vi "Get Actual Voltage.vi"(8 "error in":errorcluster, 11 "TEC 1090 in":refnum<class "Meerstetter TEC.lvclass">) -> (0 "error out":errorcluster, 2 "Number":sgl=92.92 format="%.10f", 3 "TEC 1090 out":refnum<class "Meerstetter TEC.lvclass">)   [LabVIEW 2014, in "Meerstetter Lib.lvlib" / "Meerstetter TEC.lvclass"]
uses:
  Meerstetter TEC.lvclass
  Controls/Read Parameters.ctl
  reusable/Session APIs/Serial/Serial Session.lvclass
  Meerstetter TEC.lvclass/Meerstetter TEC.ctl
  reusable/Session APIs/Serial/Public/Asynchronous Write.vi
  reusable/Session APIs/Serial/Public/Asynchronous Read.vi
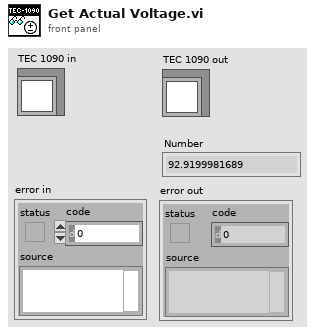
[diagram p1: front panel]
types:
  T1 = typedef "Read Parameters.ctl" = u16
  T2 = typedef "Session - Root.lvclass/Session Handle.ctl" = refnum<data-value>
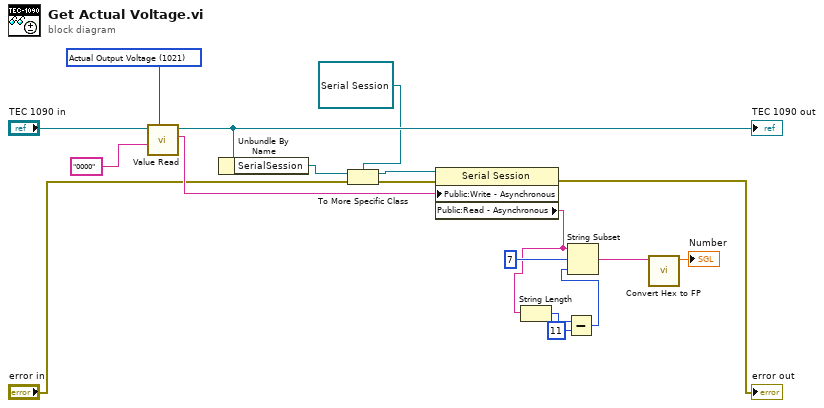
[diagram p0: block diagram]
diagram:
  w17 = T1 1021 items=["Device Type"=100, "Hardware Version"=101, "Serial Number"=102, "Firmware Version"=103, "Device Status"=104, "Error Number"=105, "Error Instance"=106, "Error Parameter"=107, "Save Data to Flash"=108, "Flash Status"=109, "Object Temperature"=1000, "Sink Temperature"=1001, "Target Obj Temperature"=1010, "Nominal Obj Temperature"=1011, "Thermal Power Mod Current"=1012, "Actual Output Current"=1020, "Actual Output Voltage"=1021, "Relative Cooling Power"=1100, "Nominal Fan Speed"=1101, "Actual Fan Speed"=1102, "Fan PWM Level"=1103, "PID Lower Limitation"=1030, "PID Upper Limitation"=1031, "PID Control Variable"=1032, "Obj Sensor Raw ADC Val"=1040, "Sink Sensor Raw ADC Val"=1041, "Object Sensor Resistance"=1042, "Sink Sensor Resistance"=1043, "Driver Input Voltage"=1060, "10V Internal Supply"=1061, "3.3V Internal Supply"=1062, "Base Plate Temperature"=1063, "Error Number"=1070, "Error Instance"=1071, "Error Parameter"=1072, "Temperature is Stable"=1200] ("Read Values")
  n1 = call "Value Read.vi"("Read Values"=w17, "Sequence"="0000", "TEC 1090"="TEC 1090 in") -> ("hex integer string"=w4:string, "TEC 1091"=w9:refnum<class "Meerstetter TEC.lvclass">)  [unwired: 7 in]
  "TEC 1090 out" <- w9
  n2 = Unbundle By Name(w9) -> ("SerialSession"=w8:T2)
  n3 = To More Specific Class(target class=refnum<data-value> refnum, reference=w8, error in="error in") -> (specific class reference=w6:refnum<data-value>, error out=w2:errorcluster)
  n4 = property class="Serial Session"(reference=w6, error in=w2, "Public:Write - Asynchronous"=w4) -> (error out=→"error out":errorcluster, "Public:Read - Asynchronous"=w5:string)  [unwired: 1 out]
  n5 = String Length(string=w5) -> (length=w13:i32)
  n6 = Subtract(x=w13, y=11) -> (x-y=w11:i32)
  n7 = String Subset(string=w5, offset (0)=7, length (rest)=w11) -> (substring=w14:string)
  n8 = call "Convert Hex to FP.vi"("Hex String In"=w14) -> ("Number"=→"Number":sgl)  [unwired: 10 in]
